vi "Cornerstone_Get.vi"(8 "error in":errorcluster, 10 "Parameter":u16(ring) items=["Wavelength", "Filter", "Grating"], 11 "VISA resource IN":refnum<visa-resource-name>) -> (0 "error out":errorcluster, 2 "Value":dbl, 3 "VISA resource OUT":refnum<visa-resource-name>)   [LabVIEW 2017]
doc: "This VI is for reading back a given parameter from the Cornerstone monochromator (grating, wavlength, filter)."
panel:
  # "Written by Kyle Montgomery, PhD\nVisit: kmontgomery.net"
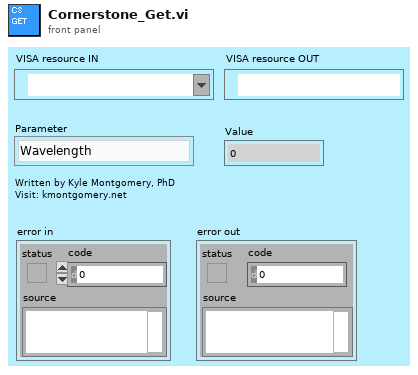
[diagram p1: front panel]
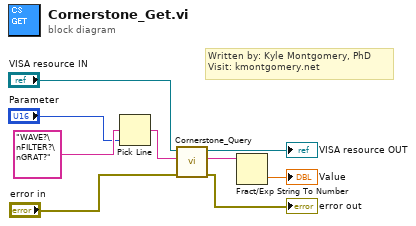
[diagram p0: block diagram]
diagram:
  # "Written by: Kyle Montgomery, PhD\nVisit: kmontgomery.net"
  n1 = Pick Line(multi-line string="WAVE?\nFILTER?\nGRAT?", line index="Parameter") -> (output string=w6:string)  [unwired: 1 out]
  n2 = call "Cornerstone_Query.vi"("error in"="error in", "Query"=w6, "VISA resource IN"="VISA resource IN") -> ("error out"=→"error out":errorcluster, "Read Data"=w1:string, "VISA resource OUT"=→"VISA resource OUT":refnum<visa-resource-name>)  [unwired: 6 out]
  n3 = Fract/Exp String To Number(string=w1) -> (number=→"Value":dbl)  [unwired: 4 out]
